vi "Log Binning.vi"(0 "Average Power":bool=TRUE, 4 "Max Freq":dbl[unit]=1000000000.0 format="%#_6p", 5 "Number Elements":u32=200, 6 "Frequencies":dbl[](array[numeric]), 7 "Spectrum":dbl[](array[numeric])) -> (2 "Frequencies Binned":dbl[](array[numeric]), 3 "Spectrum Binned":dbl[](array[numeric]))   [LabVIEW 2020]
panel:
  out "Log Range":dbl[](array[numeric])=[nan, nan, nan, nan, nan, nan, nan, nan, nan, nan, nan, nan, nan, nan, nan, nan, nan, nan, nan, nan, nan, nan, nan, nan, nan, nan, nan, nan, nan, nan, nan, nan, nan, nan, nan, nan, nan, nan, nan, nan, nan, nan, nan, nan, nan, nan, nan, nan, nan, nan, nan, nan, nan, nan, nan, nan, nan, nan, nan, nan, nan, nan, nan, nan, nan, nan, nan, nan, nan, nan, nan, nan, nan, nan, nan, nan, nan, nan, nan, nan, nan, nan, nan, nan, nan, nan, nan, nan, nan, nan, nan, nan, nan, nan, nan, nan, nan, nan, nan, nan, nan, nan, nan, nan, nan, nan, nan, nan, nan, nan, nan, nan, nan, nan, nan, nan, nan, nan, nan, nan, nan, nan, nan, nan, nan, nan, nan, nan, nan, nan, nan, nan, nan, nan, nan, nan, nan, nan, nan, nan, nan, nan, nan, nan, nan, nan, nan, nan, nan, nan, nan, nan, nan, nan, nan, nan, nan, nan, nan, nan, nan, nan, nan, nan, nan, nan, nan, nan, nan, nan, nan, nan, nan, nan, nan, nan, nan, nan, nan, nan, nan, nan, nan, nan, nan, nan, nan, nan, nan, nan, nan, nan, nan, nan, nan, nan, nan, nan, nan, nan]
  out "XY Graph":cluster{dbl[], dbl[]}[](graph)
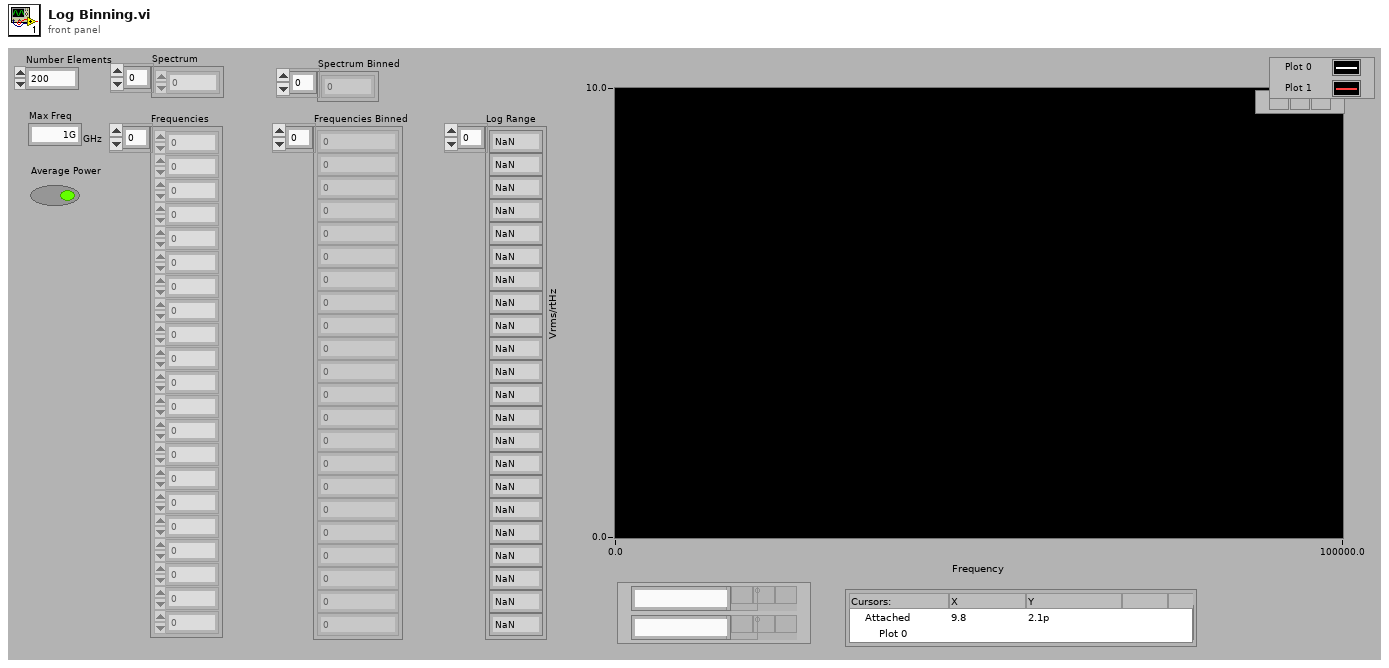
[diagram p1: front panel]
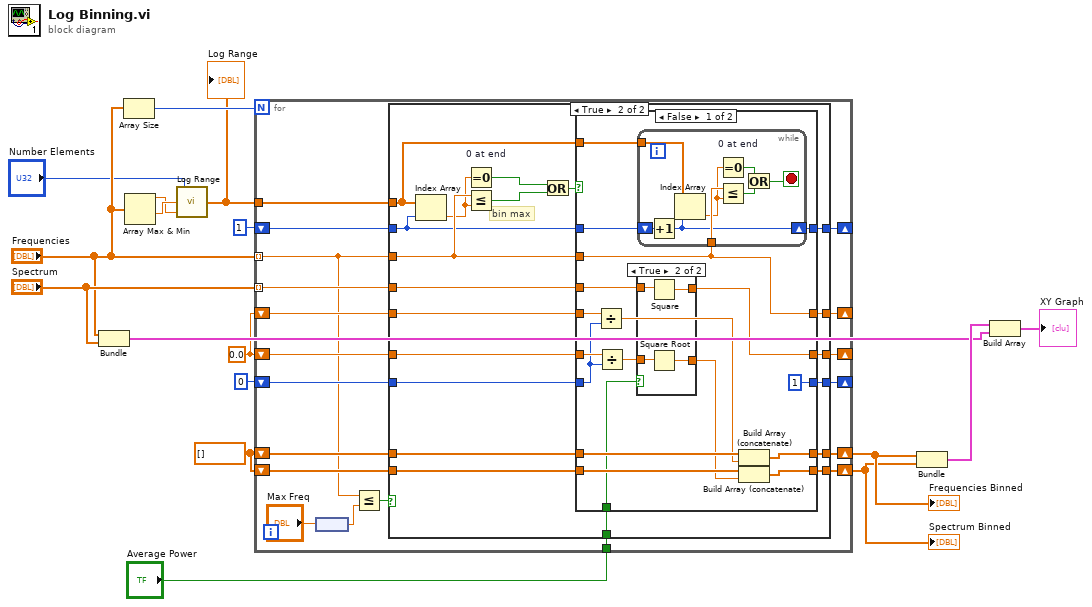
[diagram p0: block diagram]
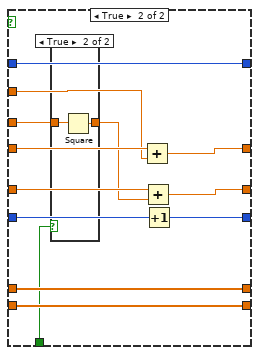
[diagram p4: hidden frame]
diagram:
  w5 = dbl[] []
  w6 = 0.0
  n1 = Bundle("Frequencies"="Frequencies", "Spectrum"="Spectrum") -> (w14:cluster{"Frequencies":dbl[], "Spectrum":dbl[]})  [unwired: 1 out]
  n2 = Array Size(array="Frequencies") -> (size(s)=w13:i32)
  n3 = Array Max & Min(array="Frequencies") -> (max value=w10:dbl, min value=w11:dbl)  [unwired: 2 out]
  n4 = call <instrlib>:"Log Range.vi"("Max"=w10, "Min"=w11, "Number Elements"="Number Elements") -> ("Log Range"=w12:dbl[])
  "Log Range" <- w12
  n5 = for {
    N: w13 -> [_]
    tunnel: "Frequencies" -> [w22] mode=indexing
    tunnel: "Spectrum" -> [w36] mode=indexing
    tunnel: w12 -> [w23]
    shift-right: [w24] -> _
    shift-left: u32 1 ("size(s)") -> [w25]
    shift-right: [w30] -> _
    shift-left: u32 0 ("size(s)") -> [w31]
    shift-right: [w34] -> _
    shift-left: w6 -> [w35]
    shift-right: [w33] -> _
    shift-left: w6 -> [w32]
    shift-right: [w29] -> w4
    shift-left: w5 -> [w28]
    shift-right: [w27] -> w3
    shift-left: w5 -> [w26]
    tunnel: "Average Power" -> [w18]
    n6 = node("Max Freq") -> (w19:dbl)
    n7 = Less Or Equal?(x=w22, y=w19) -> (x <= y?=w21:bool)
    n8 = case shown="True" w21 {
      tunnel: w22 -> [_ w62]
      tunnel: w36 -> [_ w61]
      tunnel: w35 -> [w41 w60]
      tunnel: [w41 w59] -> w34
      tunnel: [w40 w58] -> w33
      tunnel: w32 -> [w40 w57]
      tunnel: w31 -> [w39 w56]
      tunnel: [w39 w55] -> w30
      tunnel: [w38 w54] -> w29
      tunnel: w28 -> [w38 w53]
      tunnel: [w37 w52] -> w27
      tunnel: w26 -> [w37 w51]
      tunnel: w25 -> [w42 w50]
      tunnel: [w42 w49] -> w24
      tunnel: w23 -> [_ w48]
      tunnel: w18 -> [_ w43]
      frame False {
      }
      frame True {
        # "bin max"
        n9 = Index Array(array=w48, index=w50) -> (element=w44:dbl)
        n10 = Equal To 0? "0 at end"(x=w44) -> (x = 0?=w45:bool)
        n11 = Less Or Equal?(x=w62, y=w44) -> (x <= y?=w47:bool)
        n12 = Or(x=w45, y=w47) -> (x .or. y?=w46:bool)
        n13 = case shown="False" w46 {
          tunnel: w62 -> [w70 w96]
          tunnel: w61 -> [w65 w98]
          tunnel: w60 -> [w79 w107]
          tunnel: [w70 w106] -> w59
          tunnel: [w64 w105] -> w58
          tunnel: w57 -> [w78 w104]
          tunnel: w56 -> [w77 w103]
          tunnel: [u32 1 ("size(s)") w102] -> w55
          tunnel: [w76 w101] -> w54
          tunnel: w53 -> [w75 w101]
          tunnel: [w74 w100] -> w52
          tunnel: w51 -> [w73 w100]
          tunnel: w50 -> [w72 w99]
          tunnel: [w71 w99] -> w49
          tunnel: w48 -> [w69 _]
          tunnel: w43 -> [w63 w95]
          frame False {
            n14 = Divide ("Average Freq")(x=w79, y=w77) -> (x/y=w66:dbl)
            n15 = Divide ("Average Signal")(x=w78, y=w77) -> (x/y=w68:dbl)
            n16 = case shown="True" w63 {
              tunnel: w68 -> [w82 w86]
              tunnel: [w82 w85] -> w67
              tunnel: w65 -> [w81 w84]
              tunnel: [w81 w83] -> w64
              frame False {
              }
              frame True {
                n17 = Square(x=w84) -> (x^2=w83:dbl)
                n18 = Square Root(x=w86) -> (sqrt(x)=w85:dbl)
              }
            }
            n19 = while {
              tunnel: w70 -> [w93]
              tunnel: w69 -> [w92]
              shift-right: [w91] -> w71
              shift-left: w72 -> [w94]
              stop <- w88 stop-if-true
              n20 = Increment(x=w94) -> (x+1=w91:u32)
              n21 = Index Array(array=w92, index=w91) -> (element=w87:dbl)
              n22 = Equal To 0? "0 at end"(x=w87) -> (x = 0?=w89:bool)
              n23 = Less Or Equal?(x=w93, y=w87) -> (x <= y?=w90:bool)
              n24 = Or(x=w89, y=w90) -> (x .or. y?=w88:bool)
            }
            n25 = Build Array (concatenate)(w75, w66) -> (w76:dbl[])
            n26 = Build Array (concatenate)(w73, w67) -> (w74:dbl[])
          }
          frame True {
            n27 = case shown="True" w95 {
              tunnel: w98 -> [w108 w110]
              tunnel: [w108 w109] -> w97
              frame False {
              }
              frame True {
                n28 = Square(x=w110) -> (x^2=w109:dbl)
              }
            }
            n29 = Add(x=w107, y=w96) -> (x+y=w106:dbl)
            n30 = Add(x=w104, y=w97) -> (x+y=w105:dbl)
            n31 = Increment(x=w103) -> (x+1=w102:u32)
          }
        }
      }
    }
  }
  "Spectrum Binned" <- w3
  "Frequencies Binned" <- w4
  n32 = Bundle(w4, w3) -> (w17:cluster{dbl[], dbl[]})  [unwired: 1 out]
  n33 = Build Array(w17, w14) -> (→"XY Graph":cluster{"Frequencies":dbl[], "Spectrum":dbl[]}[])
